vi "Read Adjacent Containers.vi"(7 "Exclude Source":refnum<class "Message Enqueuer.lvclass">, 8 "error in (no error)":errorcluster, 11 "Transfer Line in":refnum<class "Transfer Line.lvclass">) -> (0 "error out":errorcluster, 2 "Adjacent Containers":refnum<class "Message Enqueuer.lvclass">[](array[class]), 3 "Transfer Line out":refnum<class "Transfer Line.lvclass">)   [LabVIEW 2015, in "cRIO-Carbondioxide.lvlib" / "CO2-Actor.lvlib" / "Transfer Line.lvclass"]
uses:
  Transfer Line.lvclass
  <vilib>/ActorFramework/Message Enqueuer/Message Enqueuer.lvclass
  CO2 Actor/CO2 Actor.lvclass
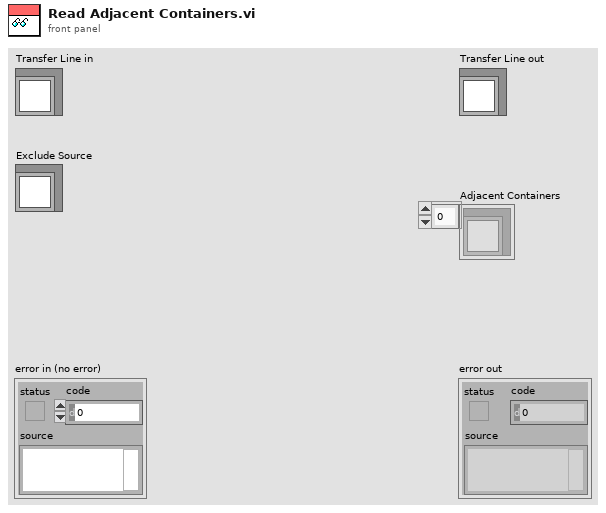
[diagram p1: front panel]
types:
  T1 = typedef "Dedicated Enqueuers.ctl" = cluster{"Freezers":cluster{"Syringe":refnum<class "Message Enqueuer.lvclass">, "Tank 1":refnum<class "Message Enqueuer.lvclass">, "Tank 2":refnum<class "Message Enqueuer.lvclass">, "Tank 3":refnum<class "Message Enqueuer.lvclass">, "Tank 4":refnum<class "Message Enqueuer.lvclass">}, "Heaters":cluster{"Syringe":refnum<class "Message Enqueuer.lvclass">, "Piston":refnum<class "Message Enqueuer.lvclass">}, "Blowers":cluster{"Tank 1":refnum<class "Message Enqueuer.lvclass">, "Tank 2":refnum<class "Message Enqueuer.lvclass">, "Tank 3":refnum<class "Message Enqueuer.lvclass">, "Tank 4":refnum<class "Message Enqueuer.lvclass">, "Syringe":refnum<class "Message Enqueuer.lvclass">}, "Sample Line":refnum<class "Message Enqueuer.lvclass">, "Storage Line":refnum<class "Message Enqueuer.lvclass">, "Transfer Line":refnum<class "Message Enqueuer.lvclass">, "Syringe Stepper":refnum<class "Message Enqueuer.lvclass">, "Syringe Line":refnum<class "Message Enqueuer.lvclass">, "Capillary Line":refnum<class "Message Enqueuer.lvclass">, "Preparation Line":refnum<class "Message Enqueuer.lvclass">, "Turbo":refnum<class "Message Enqueuer.lvclass">, "Vacuum":refnum<class "Message Enqueuer.lvclass">, "He Line":refnum<class "Message Enqueuer.lvclass">, "Cylinder":refnum<class "Message Enqueuer.lvclass">}
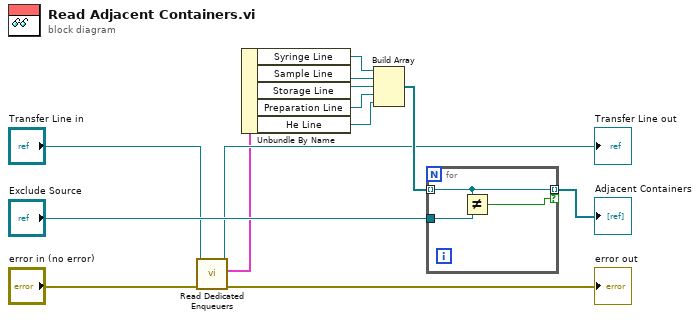
[diagram p0: block diagram]
diagram:
  n1 = call "Read Dedicated Enqueuers.vi"("error in (no error)"="error in (no error)", "CO2 Actor in"="Transfer Line in") -> ("error out"=→"error out":errorcluster, "Dedicated Enqueuers"=w2:T1, "CO2 Actor out"=→"Transfer Line out":refnum<class "Transfer Line.lvclass">)  [unwired: 6 in, 1 out]
  n2 = Unbundle By Name(w2) -> ("Syringe Line"=w3:refnum<class "Message Enqueuer.lvclass">, "Sample Line"=w12:refnum<class "Message Enqueuer.lvclass">, "Storage Line"=w5:refnum<class "Message Enqueuer.lvclass">, "Preparation Line"=w4:refnum<class "Message Enqueuer.lvclass">, "He Line"=w1:refnum<class "Message Enqueuer.lvclass">)
  n3 = Build Array(w3, w12, w5, w4, w1) -> (w10:refnum<class "Message Enqueuer.lvclass">[])
  n4 = for {
    tunnel: "Exclude Source" -> [w16]
    tunnel: w10 -> [w15] mode=indexing
    tunnel: [w15] -> w9 mode=indexing if=w14
    n5 = Not Equal?(x=w15, y=w16) -> (x != y?=w14:bool)
  }
  "Adjacent Containers" <- w9
